vi "Set DDS Sweep Stop Freq.vi"(10 "freq":dbl, 11 "channel_index":u8) -> ()   [LabVIEW 2021, in "vmmso.lvlib"]
doc: "DLL_API void WINAPI SetDDSSweepStopFreq(unsigned char channel_index, double freq);"
uses:
  vmmso.lvlib
  vmmso.dll
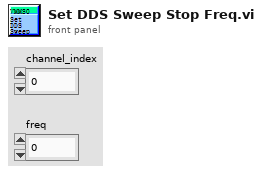
[diagram p1: front panel]
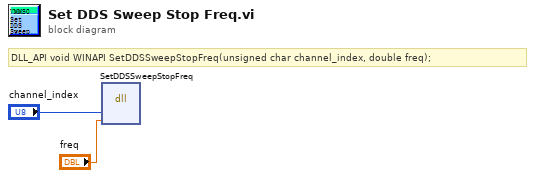
[diagram p0: block diagram]
diagram:
  # "DLL_API void WINAPI SetDDSSweepStopFreq(unsigned char channel_index, double freq);"
  n1 = dll-call lib="D:/labviewdemo/LabviewDemo 21/vmmso/vmmso.*" fn="SetDDSSweepStopFreq"("channel_index"="channel_index", "freq"="freq") -> ()  [unwired: 6 in, 2 out]
